vi "Check Default Folders.vi"(8 "error in (no error)":errorcluster, 9 "Application name":string, 10 "Application folder":path, 11 "Application Controller in":refnum<class "Application Controller.lvclass">) -> (0 "error out":errorcluster, 3 "Application Controller out":refnum<class "Application Controller.lvclass">)   [LabVIEW 2018, in "Application Controller.lvclass"]
uses:
  Application Controller.lvclass
  <vilib>/Utility/sysdir.llb/System Directory Type.ctl
  <vilib>/Utility/config.llb/Read Key (String).vi
  <vilib>/Utility/config.llb/NI_LVConfig.lvlib
panel:
  out "User temp directory":path
  out "App:Default Data Directory":path
  out "key names":string[](array[string])
  out "ini file":path
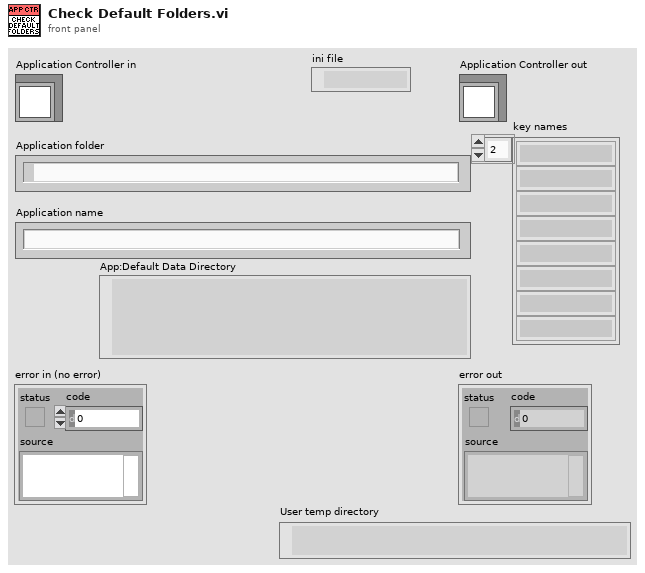
[diagram p1: front panel]
types:
  T1 = typedef "NI_LVConfig.lvlib/Config Data RefNum.ctl" = refnum<k1>
  T2 = typedef "System Directory Type.ctl" = i32
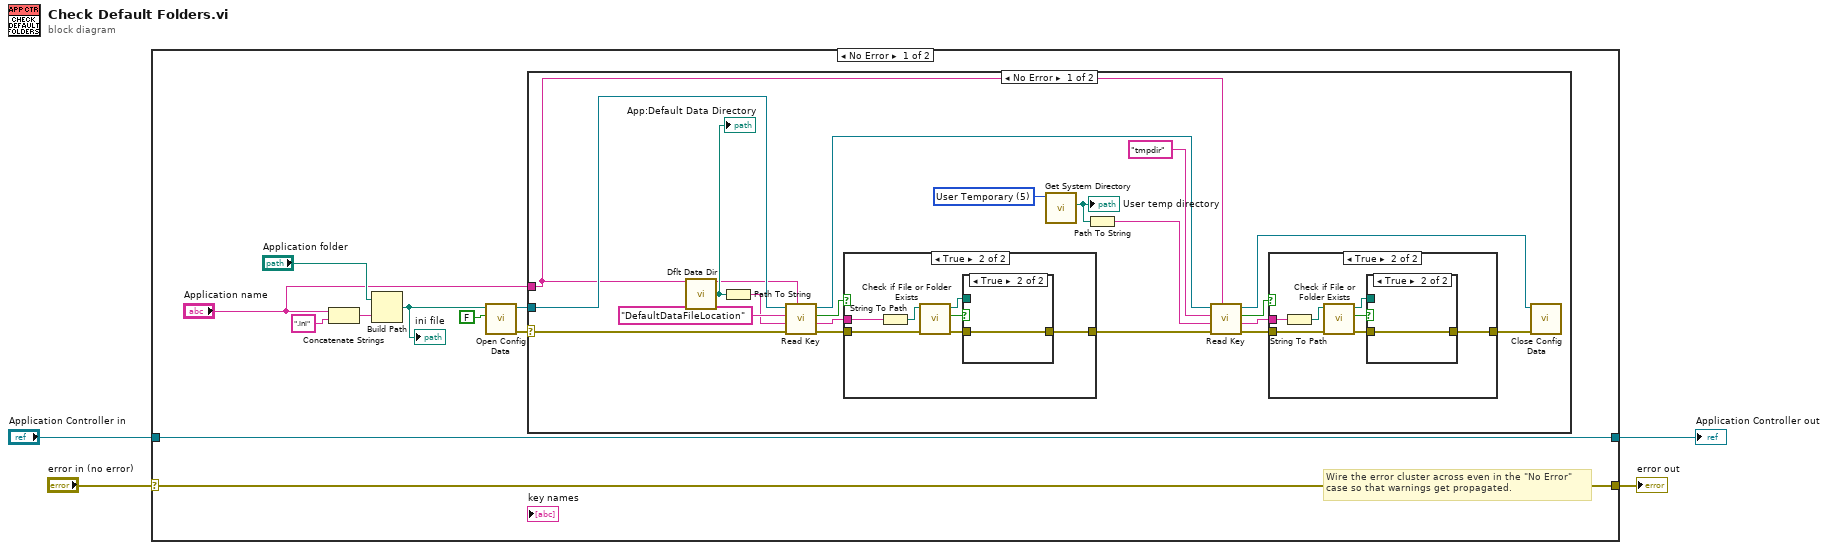
[diagram p0: block diagram]
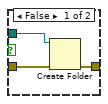
[diagram p3: hidden frame]
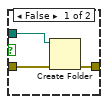
[diagram p5: hidden frame]
diagram:
  n1 = case shown="No Error" "error in (no error)" {
    selector: "error in (no error)" -> [w13 w60]
    tunnel: [w13 w60] -> w3
    tunnel: [w14 w59] -> w1
    tunnel: "Application Controller in" -> [w14 w59]
    frame No Error {
      # "Wire the error cluster across even in the \"No Error\"\ncase so that warnings get propagated."
      n2 = Concatenate Strings("Application name", ".ini" ("string")) -> (w10:string)
      n3 = Build Path(base path="Application folder", name or relative path=w10) -> (appended path=w9:path)
      "ini file" <- w9
      n4 = call <vilib>:"Open Config Data.vi"("create file if necessary (T)"=FALSE, "configuration file path"=w9) -> ("error out"=w6:errorcluster, "refnum"=w7:T1)  [unwired: 7 in, 1 out]
      n5 = case shown="No Error" w6 {
        selector: w6 -> [w33 _]
        tunnel: w7 -> [w34 _]
        tunnel: "Application name" -> [w15 _]
        frame No Error {
          w18 = T2 5 items=["User Home"=0, "User Desktop"=1, "User Documents"=2, "User Application Data"=3, "User Preferences"=4, "User Temporary"=5, "Public Documents"=6, "Public Application Data"=7, "Public Preferences"=8, "Public Cache"=13, "System Core Libraries"=9, "System Installed Libraries"=10, "Application Files"=11, "Boot Volume Root"=12] ("system directory type")
          n6 = call <vilib>:"Dflt Data Dir.vi"() -> ("App:Default Data Directory"=w31:path)
          "App:Default Data Directory" <- w31
          n7 = Path To String(path=w31) -> (string=w30:string)
          n8 = call-poly <vilib>:"Read Key.vi"("section"=w15, "error in (no error)"=w33, "default value"=w30, "key"="DefaultDataFileLocation", "refnum"=w34) -> ("error out"=w27:errorcluster, "value"=w29:string, "found?"=w28:bool, "refnum out"=w24:T1)  [unwired: 3 in]
          n9 = case shown="True" w28 {
            tunnel: w29 -> [_ w54]
            tunnel: w27 -> [w47 w52]
            tunnel: [w47 w48] -> w26
            frame False {
            }
            frame True {
              n10 = String To Path(string=w54) -> (path=w53:path)
              n11 = call <vilib>:"Check if File or Folder Exists.vi"("error in (no error)"=w52, "path"=w53) -> ("error out"=w49:errorcluster, "file or folder exists?"=w51:bool, "dup path"=w50:path)  [unwired: 7 in]
              n12 = case shown="True" w51 {
                tunnel: w50 -> [w57 _]
                tunnel: w49 -> [w56 w58]
                tunnel: [w55 w58] -> w48
                frame False {
                  n13 = Create Folder(path (use dialog)=w57, error in=w56) -> (error out=w55:errorcluster)  [unwired: 1 in, 2 out]
                }
                frame True {
                }
              }
            }
          }
          n14 = call <vilib>:"Get System Directory.vi"("system directory type"=w18) -> ("system directory"=w17:path)  [unwired: 10 in]
          "User temp directory" <- w17
          n15 = Path To String(path=w17) -> (string=w16:string)
          n16 = call-poly <vilib>:"Read Key.vi"("section"=w15, "error in (no error)"=w26, "default value"=w16, "key"="tmpdir", "refnum"=w24) -> ("error out"=w25:errorcluster, "value"=w20:string, "found?"=w19:bool, "refnum out"=w22:T1)  [unwired: 3 in]
          n17 = case shown="True" w19 {
            tunnel: w20 -> [_ w42]
            tunnel: w25 -> [w35 w40]
            tunnel: [w35 w36] -> w21
            frame False {
            }
            frame True {
              n18 = String To Path(string=w42) -> (path=w41:path)
              n19 = call <vilib>:"Check if File or Folder Exists.vi"("error in (no error)"=w40, "path"=w41) -> ("error out"=w37:errorcluster, "file or folder exists?"=w39:bool, "dup path"=w38:path)  [unwired: 7 in]
              n20 = case shown="True" w39 {
                tunnel: w38 -> [w45 _]
                tunnel: w37 -> [w44 w46]
                tunnel: [w43 w46] -> w36
                frame False {
                  n21 = Create Folder(path (use dialog)=w45, error in=w44) -> (error out=w43:errorcluster)  [unwired: 1 in, 2 out]
                }
                frame True {
                }
              }
            }
          }
          n22 = call <vilib>:"Close Config Data.vi"("error in (no error)"=w21, "refnum"=w22) -> ()  [unwired: 8 in, 2 out]
        }
        frame Error {
        }
      }
    }
    frame Error {
    }
  }
  "error out" <- w3
  "Application Controller out" <- w1
